vi "Prefix Image Name for Tree.vi"(11 "name in":string) -> (3 "name out":string)   [LabVIEW 2023]
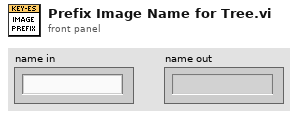
[diagram p1: front panel]
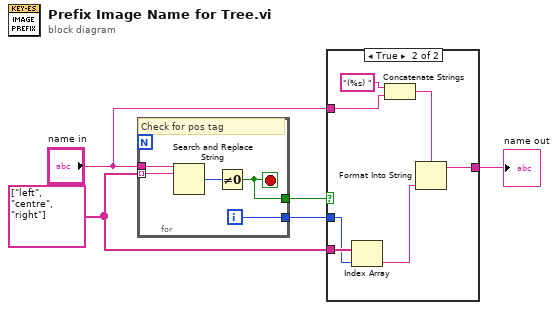
[diagram p0: block diagram]
diagram:
  w3 = string[] ["left", "centre", "right"]
  n1 = for {
    tunnel: "name in" -> [w10]
    tunnel: w3 -> [w9] mode=indexing
    tunnel: [w7] -> w4
    tunnel: [w6] -> w5
    i -> [w7]
    stop <- w6 stop-if-true
    # "Check for pos tag"
    n2 = Search and Replace String(input string=w10, search string=w9) -> (number of replacements=w8:i32)  [unwired: 6 in, 3 out]
    n3 = Not Equal To 0?(x=w8) -> (x != 0?=w6:bool)
  }
  n4 = case shown="True" w5 {
    tunnel: w4 -> [_ w17]
    tunnel: w3 -> [_ w18]
    tunnel: "name in" -> [w11 w15]
    tunnel: [w11 w12] -> w1
    frame False {
    }
    frame True {
      n5 = Index Array(array=w18, index=w17) -> (element=w13:string)
      n6 = Concatenate Strings("(%s) " ("format string"), w15) -> (w14:string)
      n7 = Format Into String(format string=w14, w13) -> (resulting string=w12:string)  [unwired: 2 in, 1 out]
    }
  }
  "name out" <- w1
